vi "TuuksSwerveWheelHeadingCalc.vi"() -> ()   [LabVIEW 2018]
panel:
  in  "DriveIn":dbl
  out "DriveOut":dbl
  out "TargetFinal":dbl
  in  "Target":dbl
  in  "Current":dbl
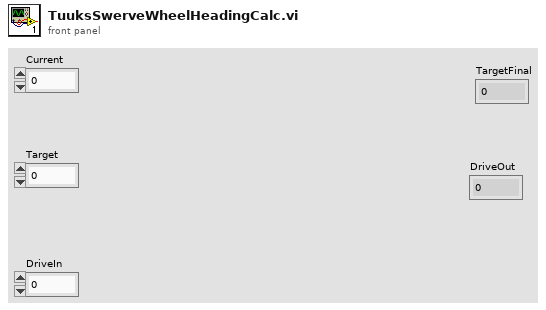
[diagram p1: front panel]
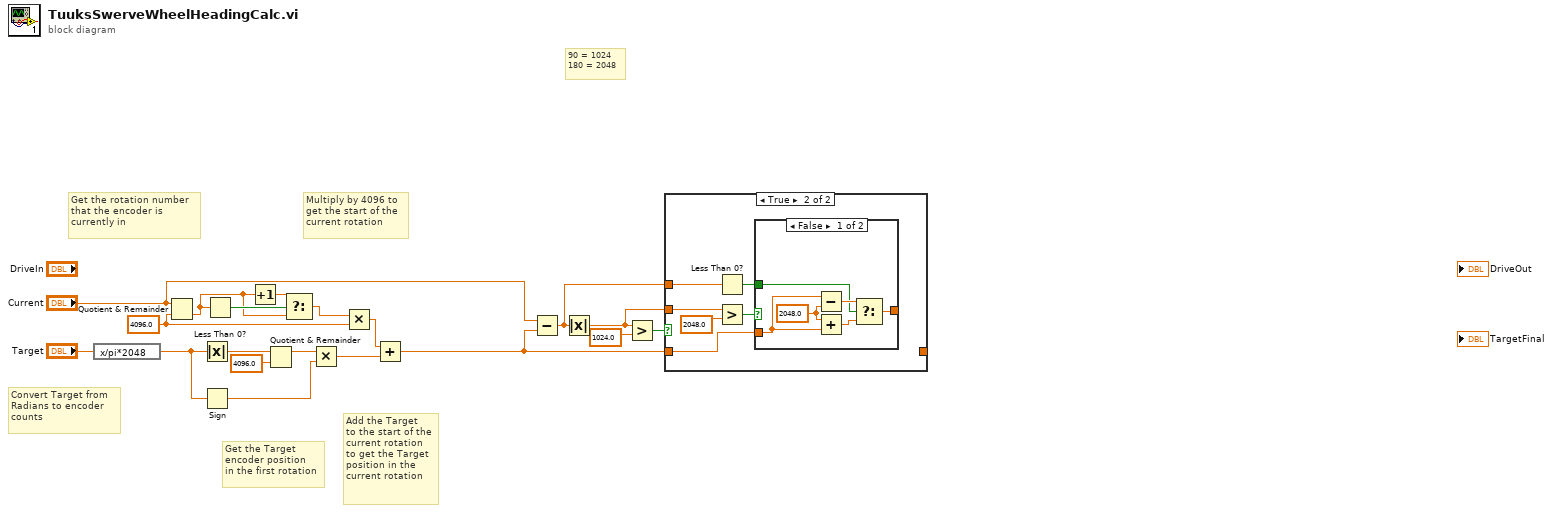
[diagram p0: block diagram]
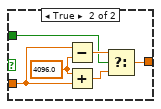
[diagram p3: hidden frame]
diagram:
  w17 = 4096.0 ("y")
  # "90 = 1024\n180 = 2048"
  # "Multiply by 4096 to\nget the start of the\ncurrent rotation"
  # "Add the Target\nto the start of the\ncurrent rotation\nto get the Target\nposition in the\ncurrent rotation"
  # "Get the Target\nencoder position\nin the first rotation"
  # "Get the rotation number\nthat the encoder is\ncurrently in"
  # "Convert Target from\nRadians to encoder\ncounts"
  n1 = expression code="x/pi*2048"("Target") -> (w8:dbl)
  n2 = Quotient & Remainder(x="Current", y=w17) -> (floor(x/y)=w11:dbl)  [unwired: 1 out]
  n3 = Absolute Value(x=w8) -> (abs(x)=w9:dbl)
  n4 = Sign(1:w8) -> (0:w7:dbl)
  n5 = Less Than 0?(x=w11) -> (x < 0?=w12:bool)
  n6 = Increment(x=w11) -> (x+1=w13:dbl)
  n7 = Quotient & Remainder(x=w9, y=4096.0) -> (x-y*floor(x/y)=w6:dbl)  [unwired: 1 out]
  n8 = Select(t=w13, s=w12, f=w11) -> (s? t:f=w10:dbl)
  n9 = Multiply(x=w6, y=w7) -> (x*y=w5:dbl)
  n10 = Multiply(x=w10, y=w17) -> (x*y=w16:dbl)
  n11 = Add(x=w16, y=w5) -> (x+y=w3:dbl)
  n12 = Subtract(x="Current", y=w3) -> (x-y=w2:dbl)
  n13 = Absolute Value(x=w2) -> (abs(x)=w1:dbl)
  n14 = Greater?(x=w1, y=1024.0) -> (0:w4:bool)
  n15 = case shown="True" w4 {
    tunnel: w3 -> [w20 w23]
    tunnel: [w20 _] -> _
    tunnel: w1 -> [_ w21]
    tunnel: w2 -> [_ w22]
    frame False {
    }
    frame True {
      n16 = Less Than 0?(x=w22) -> (x < 0?=w24:bool)
      n17 = Greater?(x=w21, y=2048.0) -> (0:w25:bool)
      n18 = case shown="False" w25 {
        tunnel: w23 -> [w28 w37]
        tunnel: w24 -> [w27 w34]
        tunnel: [w29 w33] -> _
        frame False {
          w32 = 2048.0 ("x")
          n19 = Subtract(x=w28, y=w32) -> (x-y=w30:dbl)
          n20 = Add(x=w32, y=w28) -> (x+y=w31:dbl)
          n21 = Select(t=w30, s=w27, f=w31) -> (s? t:f=w29:dbl)
        }
        frame True {
          w38 = 4096.0 ("y")
          n22 = Subtract(x=w37, y=w38) -> (x-y=w36:dbl)
          n23 = Add(x=w38, y=w37) -> (x+y=w35:dbl)
          n24 = Select(t=w36, s=w34, f=w35) -> (s? t:f=w33:dbl)
        }
      }
    }
  }
